vi "Handle Error.vi"(8 "error in (no error)":errorcluster, 11 "Network Stream in":refnum<class "Network Stream.lvclass">) -> (0 "error out":errorcluster, 2 "stop actor?":bool=TRUE, 3 "Network Stream out":refnum<class "Network Stream.lvclass">)   [LabVIEW 2014, in "Network Stream.lvlib" / "Network Stream.lvclass"]
doc: "(<B>Filename</B>: Actor Framework.lvlib:Actor.lvclass:Handle Error.vi)\n\nDefines how the actor handles an error that occurred while processing a message. By default, this method does nothing except stop the actor."
uses:
  Network Stream.lvclass
  Proxy/Proxy/Proxy.lvclass
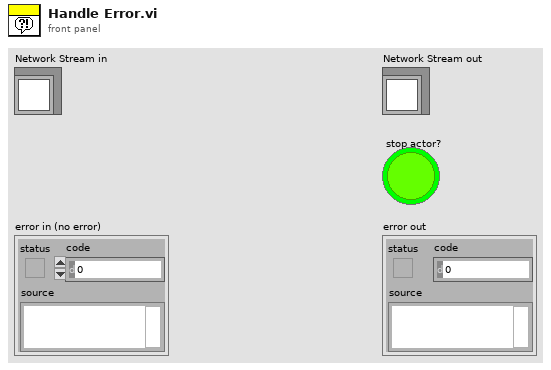
[diagram p1: front panel]
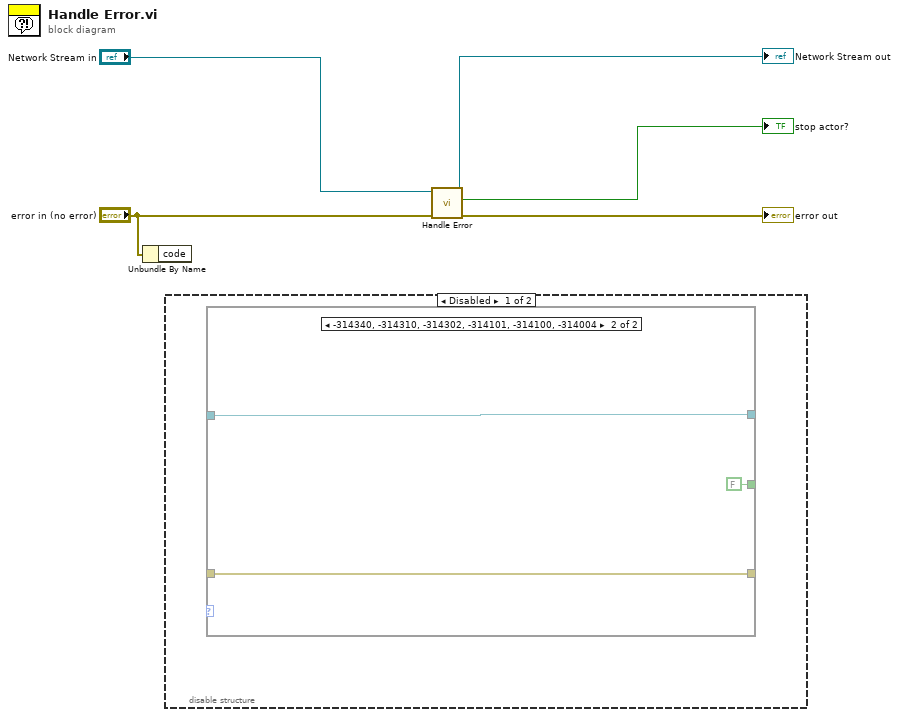
[diagram p0: block diagram]
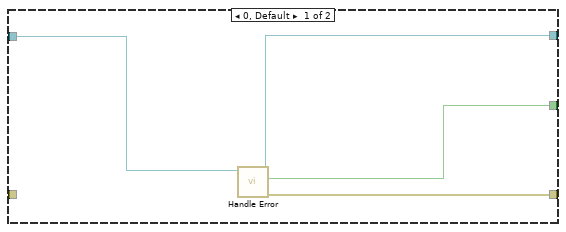
[diagram p2: hidden frame]
diagram:
  n1 = Unbundle By Name("error in (no error)") -> ()  [unwired: 1 out]
  n2 = disable-structure shown="Disabled" {
    frame Disabled {
      n3 = case shown="-314340, -314310, -314302, -314101, -314100, -314004" {
        selector: _ -> [_ _]
        tunnel: [w7 w10] -> _
        tunnel: [w9 w11] -> _
        tunnel: [w8 FALSE ("stop actor?")] -> _
        tunnel: _ -> [w6 w11]
        tunnel: _ -> [_ w10]
        frame 0, Default {
          n4 = call-parent "Handle Error.vi"("Actor in"=w6) -> ("error out"=w7:errorcluster, "stop actor?"=w8:bool, "Actor out"=w9:refnum<class "Network Stream.lvclass">)  [unwired: 8 in]
        }
        frame -314340, -314310, -314302, -314101, -314100, -314004 {
        }
      }
    }
    frame Enabled {
    }
  }
  n5 = call-parent "Handle Error.vi"("error in (no error)"="error in (no error)", "Actor in"="Network Stream in") -> ("error out"=→"error out":errorcluster, "stop actor?"=→"stop actor?":bool, "Actor out"=→"Network Stream out":refnum<class "Network Stream.lvclass">)  [unwired: 7 in]
